vi "MeasuringDevice.Init.vi"(8 "error in (no error)":errorcluster, 11 "SMU.Keithley2600":refnum<class "SMU.Keithley2600.lvclass">) -> (0 "error out":errorcluster, 3 "SMU.Keithley2600 out":refnum<class "SMU.Keithley2600.lvclass">)   [LabVIEW 2017, in "SMU.Keithley2600.lvclass"]
doc: "---------------------------------------------------------------\nJKI State Machine Objects™\nhttp://jki.net/state-machine-objects/\nCopyright (C) 2005-2015, JKI <info@jki.net>\nALL RIGHTS RESERVEDJKI State Machine Objects (SMO) 1.0.0.5\nJKI - JKI\nCopyright (c) 2016, JKI"
uses:
  SMU.Keithley2600.lvclass
  Typedefs/Resource--Cluster.ctl
  <instrlib>/Keithley 2600 Series/Public/Channel.ctl
  SMU/SMU.lvclass
  <instrlib>/Keithley 2600 Series/Keithley 2600 Series.lvlib
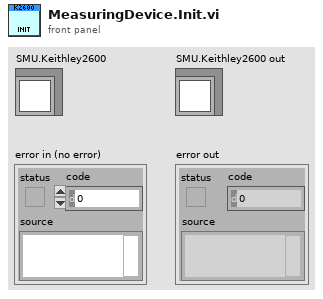
[diagram p1: front panel]
types:
  T1 = typedef "SMU.Keithley2600.lvclass/Resource--Cluster.ctl" = cluster{"VISA resource":refnum<visa-resource-name>, "Node":string, "Channel":T2}
  T2 = typedef "Keithley 2600 Series.lvlib/Channel.ctl" = enum32{"Channel A", "Channel B"}
  T3 = typedef "SMU.lvclass/Configuration--Cluster.ctl" = cluster{"VISA Resource":string, "Channel":string}
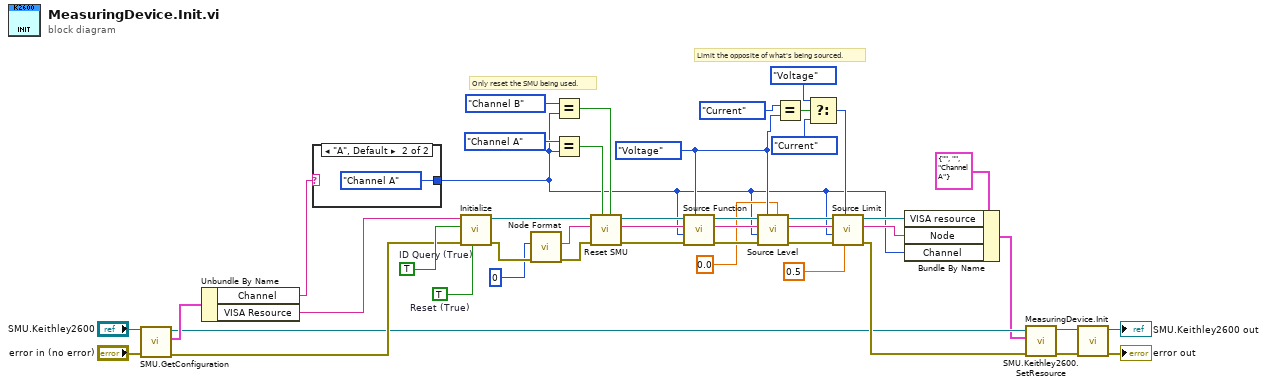
[diagram p0: block diagram]
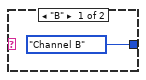
[diagram p2: hidden frame]
diagram:
  w21 = enum32{"Current", "Voltage"}."Voltage" ("Source Function (Current)")
  w15 = TRUE  # Reset (True)
  w14 = TRUE  # ID Query (True)
  # "Limit the opposite of what's being sourced."
  # "Only reset the SMU being used."
  n1 = call-dynamic "SMU.GetConfiguration.vi"("error in (no error)"="error in (no error)", "SMU"="SMU.Keithley2600") -> ("error out"=w12:errorcluster, "Configuration"=w41:T3, "SMU out"=w8:refnum<class "SMU.Keithley2600.lvclass">)  [unwired: 7 in]
  n2 = Unbundle By Name(w41) -> ("Channel"=w1:string, "VISA Resource"=w2:string)
  n3 = case shown="\"A\", Default" w1 {
    tunnel: [enum32{"Channel A", "Channel B"}."Channel B" ("x") enum32{"Channel A", "Channel B"}."Channel A" ("x")] -> w4
    frame "B" {
    }
    frame "A", Default {
    }
  }
  n4 = call <instrlib>:"Initialize.vi"("Reset (True)"=w15, "error in (no error)"=w12, "ID Query (True)"=w14, "VISA resource name"=w2) -> ("error out"=w38:errorcluster, "VISA resource name out"=w23:refnum<visa-resource-name>)  [unwired: 2 in, 4 out]
  n5 = call <instrlib>:"Node Format.vi"("error in"=w38, "Node (0-64)"=i8 0) -> ("error out"=w39:errorcluster, "Formatted Node"=w37:string)  [unwired: 8 out]
  n6 = Equal?(x=enum32{"Channel A", "Channel B"}."Channel B", y=w4) -> (x = y?=w25:bool)
  n7 = Equal?(x=enum32{"Channel A", "Channel B"}."Channel A", y=w4) -> (x = y?=w24:bool)
  n8 = call <instrlib>:"Reset SMU.vi"("SMU B (No)"=w25, "SMU A (No)"=w24, "error in (no error)"=w39, "Node In"=w37, "VISA resource name"=w23) -> ("error out"=w26:errorcluster, "Node Out"=w28:string, "VISA resource name out"=w27:refnum<visa-resource-name>)  [unwired: 4 out]
  n9 = call <instrlib>:"Source Function.vi"("Function (Current)"=w21, "error in (no error)"=w26, "Channel (Channel A)"=w4, "Node In"=w28, "VISA resource name"=w27) -> ("error out"=w31:errorcluster, "Node Out"=w29:string, "VISA resource name out"=w30:refnum<visa-resource-name>)  [unwired: 4 out]
  n10 = call <instrlib>:"Source Level.vi"("Level (0.000)"=0.0 ("Voltage start, V"), "Function (Current)"=w21, "error in (no error)"=w31, "Channel (Channel A)"=w4, "Node In"=w29, "VISA resource name"=w30) -> ("error out"=w32:errorcluster, "Node Out"=w34:string, "VISA resource name out"=w33:refnum<visa-resource-name>)  [unwired: 3 out]
  n11 = Equal?(x=enum32{"Current", "Voltage"}."Current", y=w21) -> (x = y?=w35:bool)
  n12 = Select(t=enum32{"Current", "Voltage"}."Voltage" ("x"), s=w35, f=enum32{"Current", "Voltage"}."Current") -> (s? t:f=w36:enum32{"Current", "Voltage"})
  n13 = call <instrlib>:"Source Limit.vi"("Limit (0.000)"=0.5 ("Current limit, A"), "Function (Current)"=w36, "error in (no error)"=w32, "Channel (Channel A)"=w4, "Node In"=w34, "VISA resource name"=w33) -> ("error out"=w9:errorcluster, "Node Out"=w5:string, "VISA resource name out"=w6:refnum<visa-resource-name>)  [unwired: 3 out]
  n14 = Bundle By Name(cluster=T1 {"VISA resource"="", "Node"="", "Channel"=enum."Channel A"} ("Resource"), "VISA resource"=w6, "Node"=w5, "Channel"=w4) -> (w3:T1)
  n15 = call "SMU.Keithley2600.SetResource.vi"("error in (no error)"=w9, "Resource"=w3, "SMU.Keithley2600 in"=w8) -> ("error out"=w10:errorcluster, "SMU.Keithley2600 out"=w11:refnum<class "SMU.Keithley2600.lvclass">)  [unwired: 7 in]
  n16 = call-parent "MeasuringDevice.Init.vi"("error in (no error)"=w10, "MeasuringDevice"=w11) -> ("error out"=→"error out":errorcluster, "MeasuringDevice out"=→"SMU.Keithley2600 out":refnum<class "SMU.Keithley2600.lvclass">)  [unwired: 8 in]
